vi "defects database.vi"(0 "Array 2":dbl[][](array[numeric]), 2 "table":string, 3 "pallet number":i32, 4 "curv number":i32, 5 "error in (no error)":errorcluster, 7 "condition":bool=TRUE) -> (17 "error out":errorcluster)   [LabVIEW 2019]
uses:
  <vilib>/addons/database/Auxilliary.llb/DB Tools Format Datetime String (Time Stamp).vi
  <vilib>/addons/database/NI_Database_API.lvlib
  database.lvlib
panel:
  in  "error in (no error) 2":errorcluster
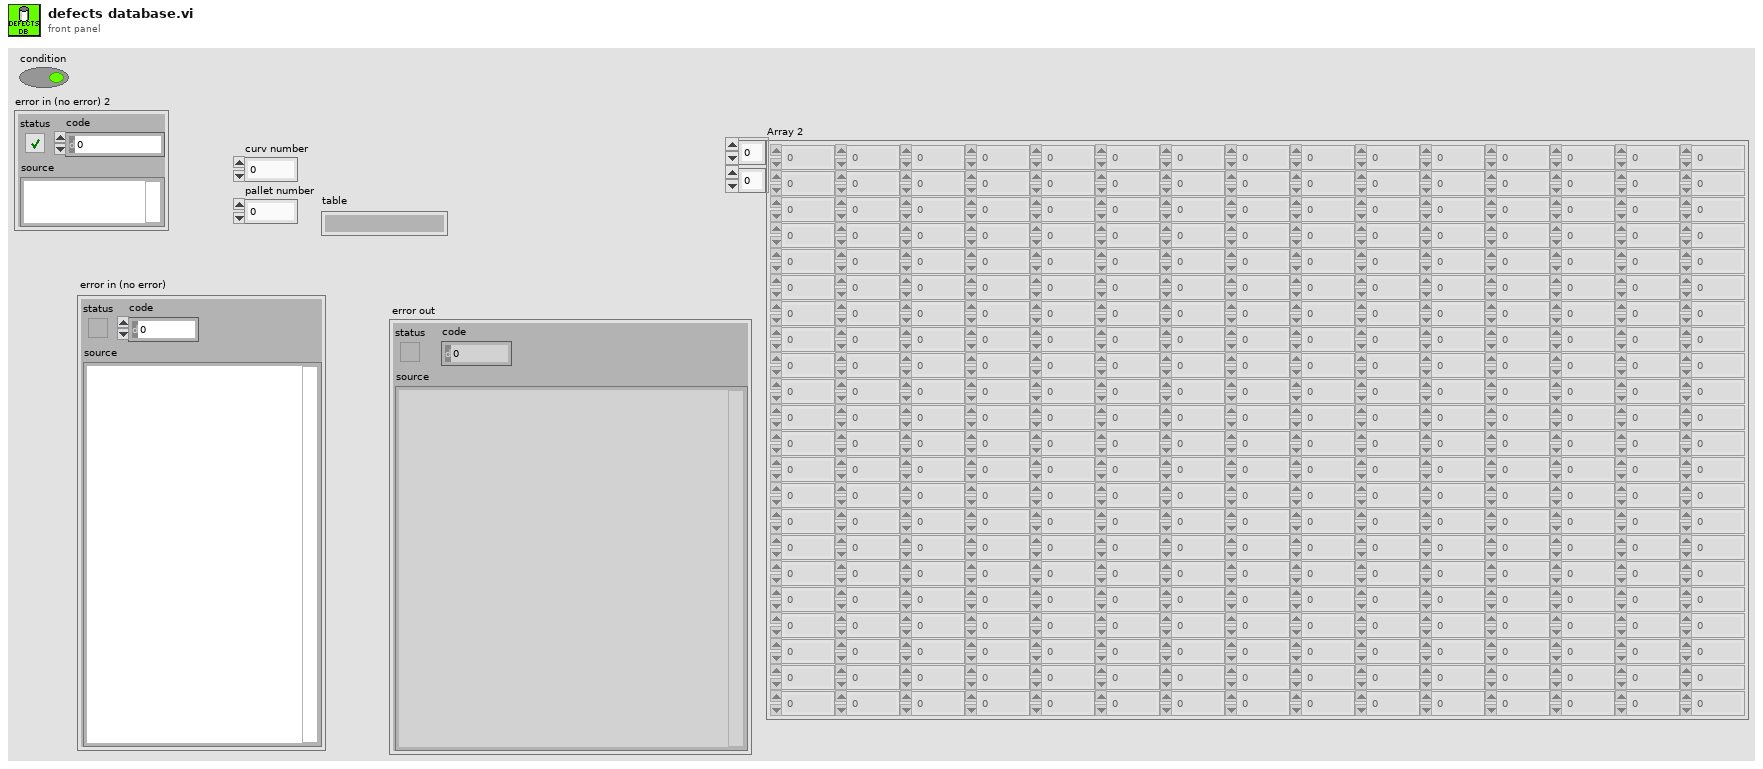
[diagram p1: front panel]
types:
  T1 = cluster{"plt number dis":i16, "Table Name":string, "Database Name":string, "DB days to save":i16, "IP #":string, "Img Path":path, "Port":u16, "time out":u16, "madule path":path, "IP # speed":string, "counting device":enum16{"Sensors", "Line Speed", "Sensors&Speed"}}
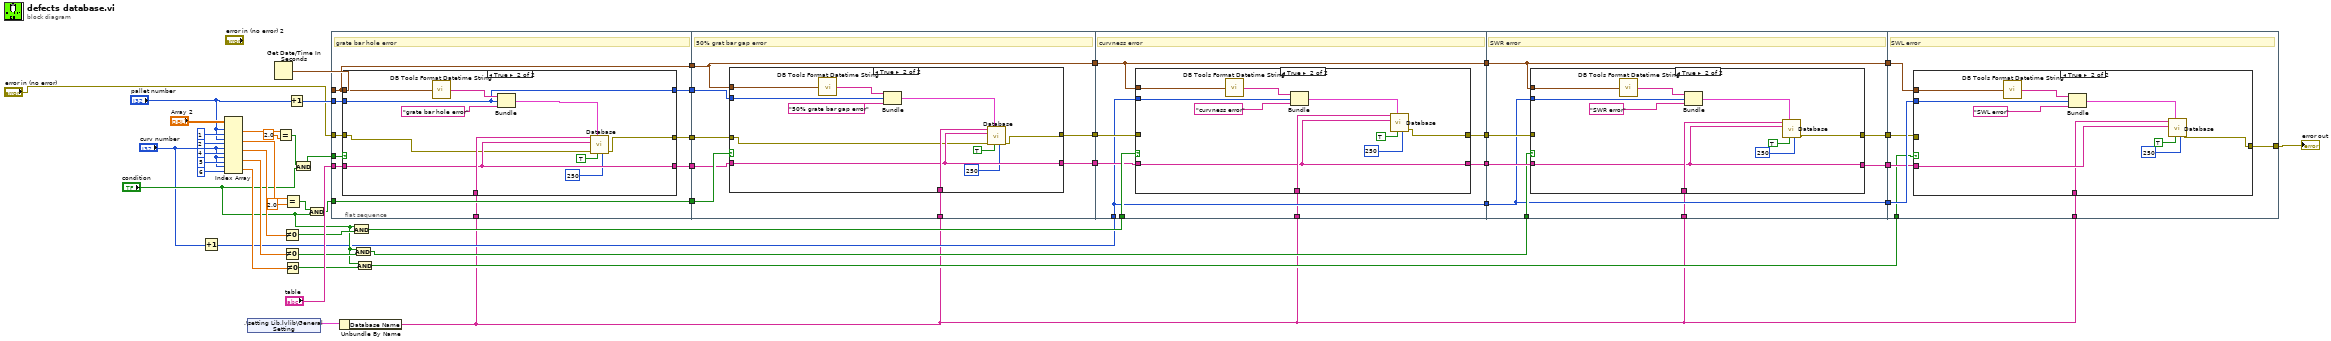
[diagram p0: block diagram]
diagram:
  n1 = Increment(x="curv number") -> (x+1=w5:i32)
  n2 = Index Array(array="Array 2", index (row) #1="pallet number", index (col) #1=1 ("disabled index (col)"), index (row) #2="pallet number", index (col) #2=2 ("disabled index (col)"), index (row) #3="curv number", index (col) #3=4 ("disabled index (col)"), index (row) #4="curv number", index (col) #4=5 ("disabled index (col)"), index (row) #5="curv number", index (col) #5=6 ("disabled index (col)")) -> (element #1=w47:dbl, element #2=w43:dbl, element #3=w35:dbl, element #4=w25:dbl, element #5=w24:dbl)
  n3 = shared-variable ".\\setting Lib.lvlib\\General Setting"() -> (w2:T1)  [unwired: 1 in, 1 out]
  n4 = Get Date/Time In Seconds() -> (seconds since 1Jan1904=w50:timestamp)
  n5 = Equal?(x=w47, y=2.0) -> (x = y?=w19:bool)
  n6 = Not Equal To 0?(x=w35) -> (x != 0?=w15:bool)
  n7 = Not Equal To 0?(x=w25) -> (x != 0?=w13:bool)
  n8 = Not Equal To 0?(x=w24) -> (x != 0?=w10:bool)
  n9 = Equal?(x=w43, y=2.0) -> (x = y?=w17:bool)
  n10 = Increment(x="pallet number") -> (x+1=w7:i32)
  n11 = And(x=w19, y="condition") -> (x .and. y?=w18:bool)
  n12 = And(x=w17, y="condition") -> (x .and. y?=w16:bool)
  n13 = flat-sequence {
    tunnel: w50 -> [w54]
    tunnel: w7 -> [w60]
    tunnel: "table" -> [w59]
    tunnel: w18 -> [w58]
    tunnel: [w57] -> w41
    tunnel: w16 -> [w57]
    tunnel: [w56] -> w40
    tunnel: [w55] -> w39
    tunnel: [w54] -> w38
    tunnel: [w53] -> w33
    tunnel: "error in (no error)" -> [w52]
    tunnel: w1 -> [w51]
    tunnel: w41 -> [w82]
    tunnel: w40 -> [w81]
    tunnel: w39 -> [w80]
    tunnel: w38 -> [w79]
    tunnel: [w79] -> w37
    tunnel: [w78] -> w34
    tunnel: w33 -> [w77]
    tunnel: [w76] -> w32
    tunnel: w1 -> [w75]
    tunnel: w37 -> [w100]
    tunnel: w14 -> [w103]
    tunnel: w34 -> [w102]
    tunnel: w5 -> [w99]
    tunnel: w32 -> [w101]
    tunnel: [w100] -> w31
    tunnel: [w99] -> w30
    tunnel: [w98] -> w29
    tunnel: [w97] -> w28
    tunnel: w1 -> [w96]
    tunnel: w31 -> [w120]
    tunnel: w30 -> [w119]
    tunnel: w29 -> [w123]
    tunnel: w28 -> [w122]
    tunnel: w12 -> [w121]
    tunnel: [w120] -> w23
    tunnel: [w119] -> w22
    tunnel: [w118] -> w21
    tunnel: [w117] -> w20
    tunnel: w1 -> [w116]
    tunnel: w23 -> [w142]
    tunnel: w22 -> [w141]
    tunnel: w21 -> [w140]
    tunnel: w20 -> [w139]
    tunnel: w9 -> [w138]
    tunnel: [w137] -> w3
    tunnel: w1 -> [w136]
    frame #0 {
      # "grate bar hole error"
      n14 = case shown="True" w58 {
        tunnel: w54 -> [_ w74]
        tunnel: w60 -> [w62 w71]
        tunnel: w59 -> [w63 w68]
        tunnel: [w63 w68] -> w56
        tunnel: [w62 w71] -> w55
        tunnel: [w61 w66] -> w53
        tunnel: w52 -> [w61 w67]
        tunnel: w51 -> [_ w69]
        frame False {
        }
        frame True {
          n15 = call-poly <vilib>:"DB Tools Format Datetime String.vi"("time stamp"=w74) -> ("date/time string"=w73:string)
          n16 = Bundle("date/time string"=w73, w71, "grate bar hole error") -> (w70:cluster{"date/time string":string, i32, string})  [unwired: 1 in]
          n17 = call "Database.vi"("Maximum Row"=250, "Delete row?"=TRUE, "Data"=w70, "Error in"=w67, "Table"=w68, "Connection"=w69) -> ("Error out"=w66:errorcluster)  [unwired: 5 in]
        }
      }
    }
    frame #1 {
      # "50% grat bar gap error"
      n18 = case shown="True" w82 {
        tunnel: w79 -> [_ w95]
        tunnel: w80 -> [_ w93]
        tunnel: w81 -> [w84 w90]
        tunnel: [w84 w90] -> w78
        tunnel: w77 -> [w83 w88]
        tunnel: [w83 w87] -> w76
        tunnel: w75 -> [_ w91]
        frame False {
        }
        frame True {
          n19 = call-poly <vilib>:"DB Tools Format Datetime String.vi"("time stamp"=w95) -> ("date/time string"=w94:string)
          n20 = Bundle("date/time string"=w94, w93, "50% grate bar gap error") -> (w89:cluster{"date/time string":string, i32, string})  [unwired: 1 in]
          n21 = call "Database.vi"("Maximum Row"=250, "Delete row?"=TRUE, "Data"=w89, "Error in"=w88, "Table"=w90, "Connection"=w91) -> ("Error out"=w87:errorcluster)  [unwired: 5 in]
        }
      }
    }
    frame #2 {
      # "curvness error"
      n22 = case shown="True" w103 {
        tunnel: w100 -> [_ w115]
        tunnel: w99 -> [_ w113]
        tunnel: w102 -> [w104 w107]
        tunnel: w101 -> [w105 _]
        tunnel: [w105 w106] -> w98
        tunnel: [w104 w107] -> w97
        tunnel: w96 -> [_ w108]
        frame False {
        }
        frame True {
          n23 = call-poly <vilib>:"DB Tools Format Datetime String.vi"("time stamp"=w115) -> ("date/time string"=w114:string)
          n24 = Bundle("date/time string"=w114, w113, "curvness error") -> (w109:cluster{"date/time string":string, i32, string})  [unwired: 1 in]
          n25 = call "Database.vi"("Maximum Row"=250, "Delete row?"=TRUE, "Data"=w109, "Table"=w107, "Connection"=w108) -> ("Error out"=w106:errorcluster)  [unwired: 6 in]
        }
      }
    }
    frame #3 {
      # "SWR error"
      n26 = case shown="True" w121 {
        tunnel: w120 -> [_ w135]
        tunnel: w119 -> [_ w133]
        tunnel: w122 -> [w124 w127]
        tunnel: w123 -> [w125 _]
        tunnel: [w125 w126] -> w118
        tunnel: [w124 w127] -> w117
        tunnel: w116 -> [_ w128]
        frame False {
        }
        frame True {
          n27 = call-poly <vilib>:"DB Tools Format Datetime String.vi"("time stamp"=w135) -> ("date/time string"=w134:string)
          n28 = Bundle("date/time string"=w134, w133, "SWR error") -> (w129:cluster{"date/time string":string, i32, string})  [unwired: 1 in]
          n29 = call "Database.vi"("Maximum Row"=250, "Delete row?"=TRUE, "Data"=w129, "Table"=w127, "Connection"=w128) -> ("Error out"=w126:errorcluster)  [unwired: 6 in]
        }
      }
    }
    frame #4 {
      # "SWL error"
      n30 = case shown="True" w138 {
        tunnel: w142 -> [_ w153]
        tunnel: w141 -> [_ w151]
        tunnel: w139 -> [_ w146]
        tunnel: w140 -> [w143 _]
        tunnel: [w143 w144] -> w137
        tunnel: w136 -> [_ w145]
        frame False {
        }
        frame True {
          n31 = call-poly <vilib>:"DB Tools Format Datetime String.vi"("time stamp"=w153) -> ("date/time string"=w152:string)
          n32 = Bundle("date/time string"=w152, w151, "SWL error") -> (w147:cluster{"date/time string":string, i32, string})  [unwired: 1 in]
          n33 = call "Database.vi"("Maximum Row"=250, "Delete row?"=TRUE, "Data"=w147, "Table"=w146, "Connection"=w145) -> ("Error out"=w144:errorcluster)  [unwired: 6 in]
        }
      }
    }
  }
  n34 = Unbundle By Name(w2) -> ("Database Name"=w1:string)
  n35 = And(x="condition", y=w15) -> (x .and. y?=w14:bool)
  n36 = And(x="condition", y=w13) -> (x .and. y?=w12:bool)
  n37 = And(x="condition", y=w10) -> (x .and. y?=w9:bool)
  "error out" <- w3
